vi "CreateSampleNode.vi"(8 "Error In":errorcluster, 10 "Experiment":T1={"File Path"=path "", "Operator"="Operator", "Project"="Project Description", "Target Dose (dpa)"=0.0, "Sample"={"Name"="", "Description"="", "Molar Mass (g/mol)"=0.0, "Density (g/cm^3)"=0.0, "Irradiation Area (cm^2)"=0.0, "SRIM Damage Peak (disp * ions/cm)"=0.0}, "Beam Line"={"Type"=enum."Ion Beam Analysis", "Ion"=enum."H", "Charge State"=0, "Total Source Ion Energy (kV)"=nan}, "Runs"=[]} {"Beam Line"."Charge State" min=1}, 11 "DOM Document In":refnum<k20>) -> (0 "Error out":errorcluster, 2 "Sample Node":refnum<k20>, 3 "DOM Document Out":refnum<k20>)   [LabVIEW 2012]
uses:
  Experiment.ctl
  Sample.ctl
  BeamLine.ctl
  BeamLineType.ctl
  BeamLineIon.ctl
  ExperimentRun.ctl
  ExperimentRunTiming.ctl
  ExperimentRunDose.ctl
  ExperimentRunFluence.ctl
  ExperimentRunTotalCharge.ctl
  <resource>/objmgr/DOMUserDefRef.rc
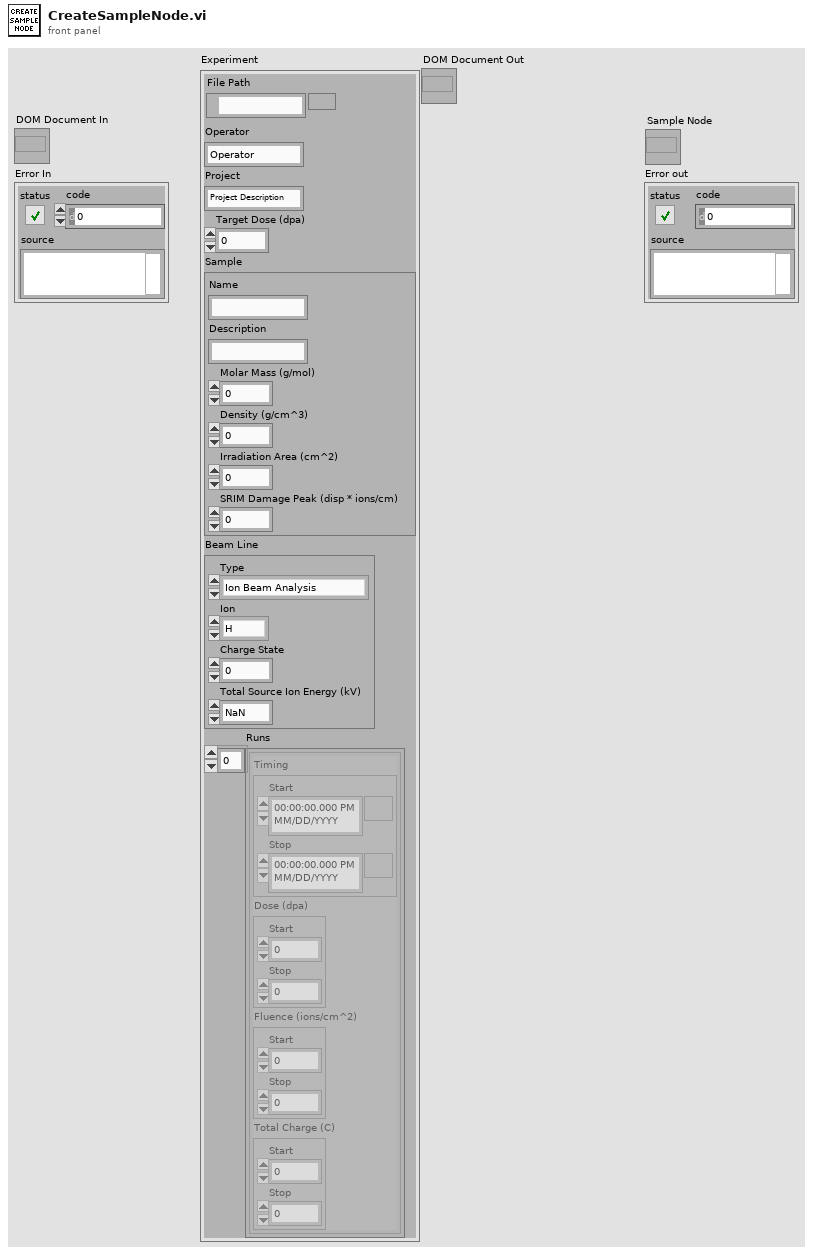
[diagram p1: front panel]
types:
  T1 = typedef "Experiment.ctl" = cluster{"File Path":path, "Operator":string, "Project":string, "Target Dose (dpa)":dbl, "Sample":T2, "Beam Line":T3, "Runs":T6[]}
  T2 = typedef "Sample.ctl" = cluster{"Name":string, "Description":string, "Molar Mass (g/mol)":dbl, "Density (g/cm^3)":dbl, "Irradiation Area (cm^2)":dbl, "SRIM Damage Peak (disp * ions/cm)":dbl}
  T3 = typedef "BeamLine.ctl" = cluster{"Type":T4, "Ion":T5, "Charge State":u8, "Total Source Ion Energy (kV)":dbl}
  T4 = typedef "BeamLineType.ctl" = enum16{"Ion Beam Analysis", "Auxiliary", "Radiation Damage"}
  T5 = typedef "BeamLineIon.ctl" = enum16{"H", "He", "C", "Fe", "Ni", "Pt", "Si", "Ag", "Au"}
  T6 = typedef "ExperimentRun.ctl" = cluster{"Timing":T7, "Dose (dpa)":T8, "Fluence (ions/cm^2)":T9, "Total Charge (C)":T10}
  T7 = typedef "ExperimentRunTiming.ctl" = cluster{"Start":timestamp, "Stop":timestamp}
  T8 = typedef "ExperimentRunDose.ctl" = cluster{"Start":dbl, "Stop":dbl}
  T9 = typedef "ExperimentRunFluence.ctl" = cluster{"Start":dbl, "Stop":dbl}
  T10 = typedef "ExperimentRunTotalCharge.ctl" = cluster{"Start":dbl, "Stop":dbl}
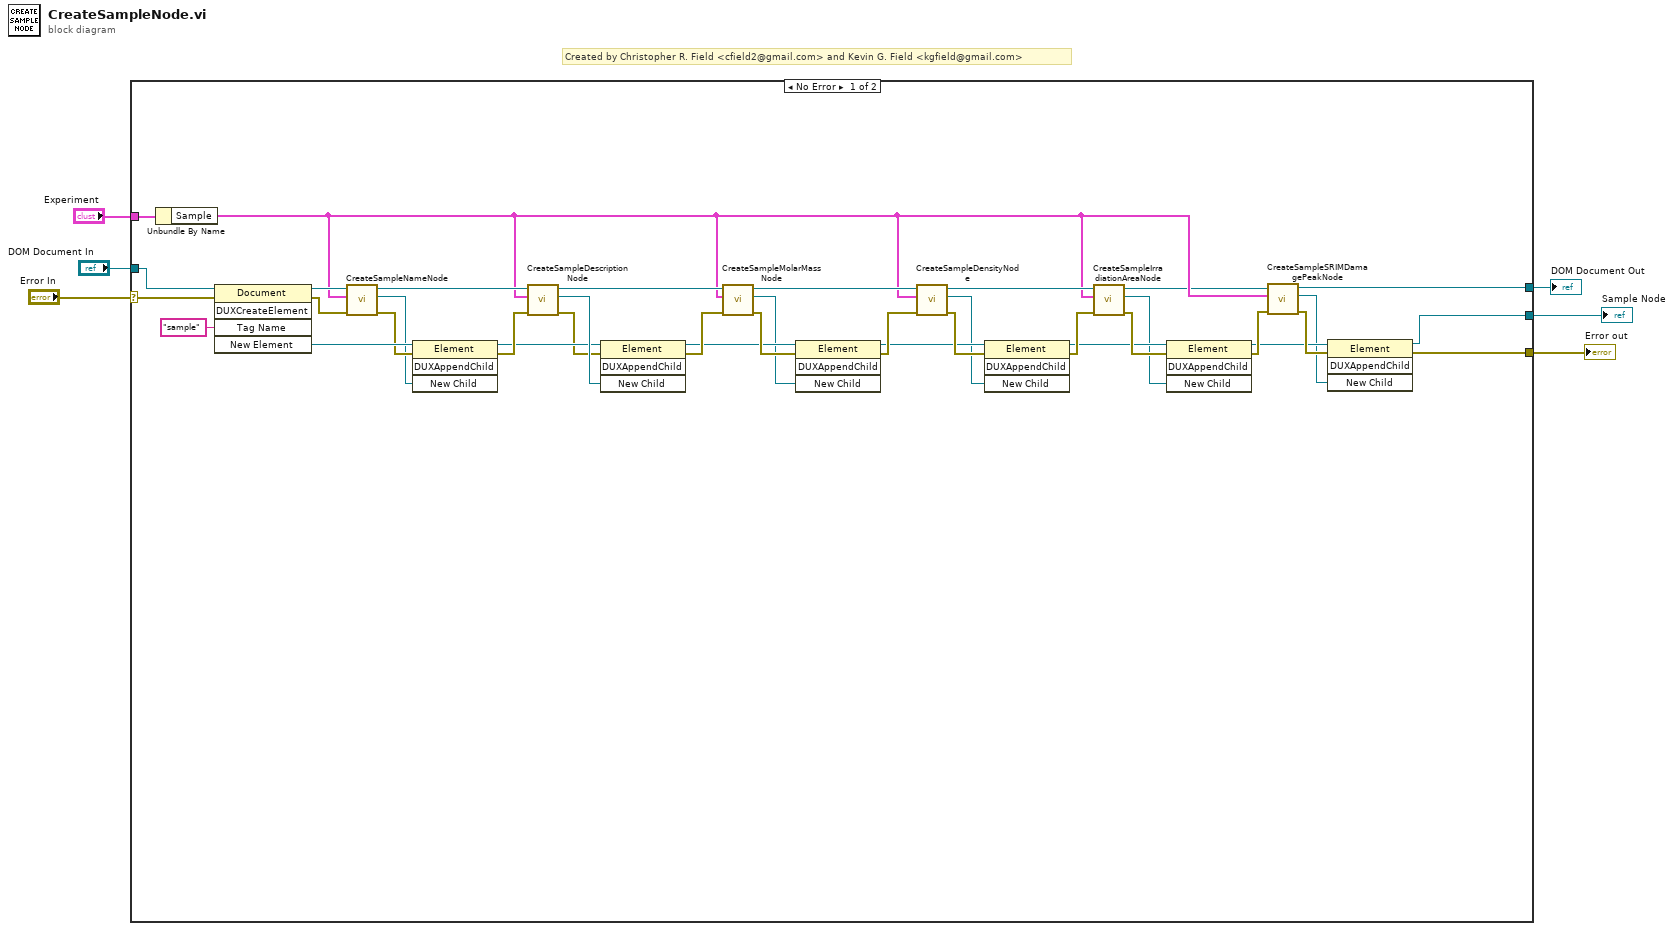
[diagram p0: block diagram]
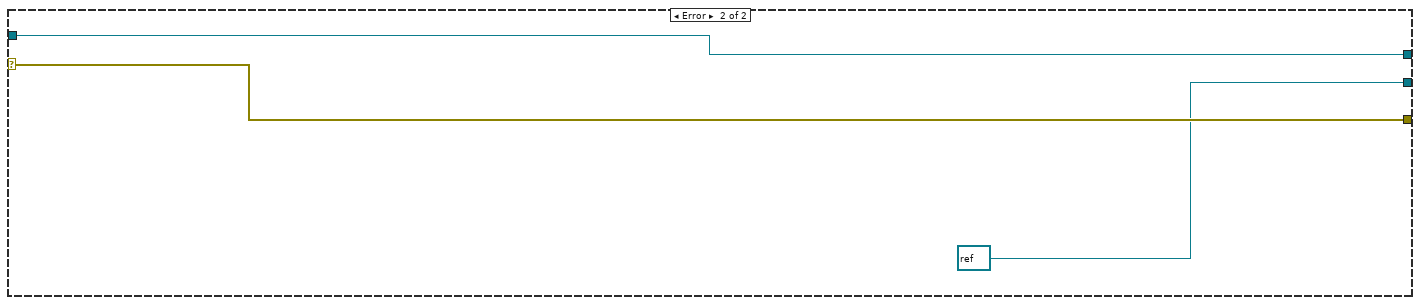
[diagram p2: hidden frame]
diagram:
  # "Created by Christopher R. Field <cfield2@gmail.com> and Kevin G. Field <kgfield@gmail.com>"
  n1 = case shown="No Error" "Error In" {
    selector: "Error In" -> [w41 w46]
    tunnel: "DOM Document In" -> [w44 w47]
    tunnel: [w7 refnum<k20> refnum ("Operator Node 2")] -> w5
    tunnel: [w16 w46] -> w4
    tunnel: "Experiment" -> [w42 _]
    tunnel: [w24 w47] -> w1
    frame No Error {
      n2 = Unbundle By Name(w42) -> ("Sample"=w26:T2)
      n3 = invoke class="Document" method="DUXCreateElement"(reference=w44, error in=w41, "Tag Name"="sample") -> (reference out=w40:refnum<k20>, error out=w39:errorcluster, "New Element"=w38:refnum<k20>)  [unwired: 2 in, 2 out]
      n4 = call "CreateSampleNameNode.vi"("Error In"=w39, "Sample"=w26, "DOM Document In"=w40) -> ("Error out"=w37:errorcluster, "Sample Name Node"=w36:refnum<k20>, "DOM Document Out"=w35:refnum<k20>)  [unwired: 6 in]
      n5 = invoke class="Element" method="DUXAppendChild"(reference=w38, error in=w37, "New Child"=w36) -> (reference out=w32:refnum<k20>, error out=w34:errorcluster)  [unwired: 1 in, 2 out]
      n6 = call "CreateSampleDescriptionNode.vi"("Error In"=w34, "Sample"=w26, "DOM Document In"=w35) -> ("Error out"=w31:errorcluster, "Sample Description Node"=w33:refnum<k20>, "DOM Document Out"=w30:refnum<k20>)  [unwired: 6 in]
      n7 = invoke class="Element" method="DUXAppendChild"(reference=w32, error in=w31, "New Child"=w33) -> (reference out=w15:refnum<k20>, error out=w29:errorcluster)  [unwired: 1 in, 2 out]
      n8 = call "CreateSampleMolarMassNode.vi"("Error In"=w29, "Sample"=w26, "DOM Document In"=w30) -> ("Error out"=w23:errorcluster, "Sample Molar Mass Node"=w11:refnum<k20>, "DOM Document Out"=w28:refnum<k20>)  [unwired: 6 in]
      n9 = invoke class="Element" method="DUXAppendChild"(reference=w15, error in=w23, "New Child"=w11) -> (reference out=w14:refnum<k20>, error out=w22:errorcluster)  [unwired: 1 in, 2 out]
      n10 = call "CreateSampleDensityNode.vi"("Error In"=w22, "Sample"=w26, "DOM Document In"=w28) -> ("Error out"=w21:errorcluster, "Sample Density Node"=w10:refnum<k20>, "DOM Document Out"=w27:refnum<k20>)  [unwired: 6 in]
      n11 = invoke class="Element" method="DUXAppendChild"(reference=w14, error in=w21, "New Child"=w10) -> (reference out=w13:refnum<k20>, error out=w20:errorcluster)  [unwired: 1 in, 2 out]
      n12 = call "CreateSampleIrradiationAreaNode.vi"("Error In"=w20, "Sample"=w26, "DOM Document In"=w27) -> ("Error out"=w19:errorcluster, "Sample Irradiation Area Node"=w9:refnum<k20>, "DOM Document Out"=w25:refnum<k20>)  [unwired: 6 in]
      n13 = invoke class="Element" method="DUXAppendChild"(reference=w13, error in=w19, "New Child"=w9) -> (reference out=w12:refnum<k20>, error out=w18:errorcluster)  [unwired: 1 in, 2 out]
      n14 = call "CreateSampleSRIMDamagePeakNode.vi"("Error In"=w18, "Sample"=w26, "DOM Document In"=w25) -> ("Error out"=w17:errorcluster, "Sample SRIM Damage Peak Node"=w8:refnum<k20>, "DOM Document Out"=w24:refnum<k20>)  [unwired: 6 in]
      n15 = invoke class="Element" method="DUXAppendChild"(reference=w12, error in=w17, "New Child"=w8) -> (reference out=w7:refnum<k20>, error out=w16:errorcluster)  [unwired: 1 in, 2 out]
    }
    frame Error {
    }
  }
  "Sample Node" <- w5
  "Error out" <- w4
  "DOM Document Out" <- w1
